vi "send and receive.vi"(6 "timeout (25000ms)":i32=25000, 8 "error in (no error)":errorcluster, 9 "data":string, 10 "command":string, 11 "daemon reference in":refnum<k5>) -> (0 "error out":errorcluster, 2 "response":string, 3 "daemon reference out":refnum<k5>)   [LabVIEW 2017]
doc: "This command is used by the API to send and receive a response from the Daemon.\n------------------------------------------\nDyLab - Network QMH Architecture 1.0.0.33\nDyson Technology Ltd Copyright (c) 2022, Dyson Technology Ltd\n____________________________________________\nDIPC 692 Daemon API 7.0.0.1\nSam Tee - Dyson Technology Ltd\nCopyright (c) 2024, Dyson Technology Ltd"
panel:
  out "Numeric":i32
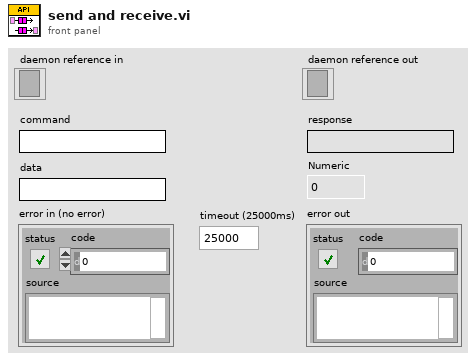
[diagram p1: front panel]
types:
  T1 = typedef "HD Config.ctl" = cluster{" PC":cluster{"PC Address":u8[], "PC Port":i32}, "FCO":cluster{"COM":refnum<visa-resource-name>, "Baudrate":u32}, "DC Power ":cluster{"COM":refnum<visa-resource-name>, "Baudrate":u32}, "PW3336":cluster{"COM":refnum<visa-resource-name>, "Baudrate":u32}, "Lefoo":cluster{"COM":refnum<visa-resource-name>, "Baudrate":u32}, "AI Model":cluster{"COM":refnum<visa-resource-name>, "Baudrate":u32}, "DIPC":cluster{"COM":refnum<visa-resource-name>}, "RFID":cluster{"IP Address":string, "Port":u16, "Retry":u16}, "Motor":cluster{"COM":refnum<visa-resource-name>, "Baudrate":u32}, "Fail_resume_mode":bool, "GRR":bool}
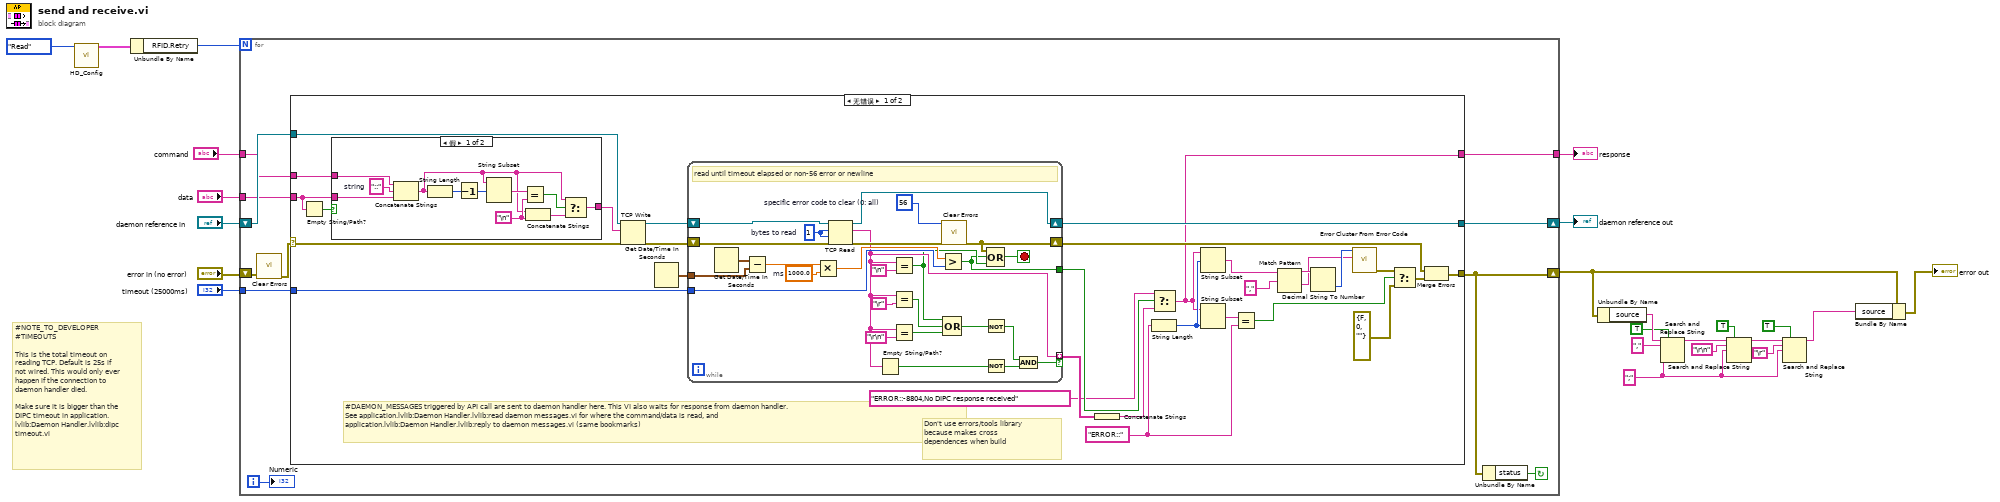
[diagram p0: block diagram]
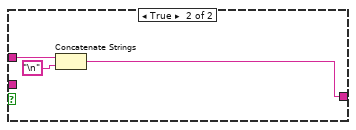
[diagram p2: hidden frame]
diagram:
  w1 = ";" ("替换字符串(\"\")")
  # "#NOTE_TO_DEVELOPER \n#TIMEOUTS\n\nThis is the total timeout on reading TCP. Default is 25s if not wired. This would only ever happen if the connection to daemon handler died.\n\nMake sure it is bigger than the DIPC timeout in application.lvlib:Daemon Handler.lvlib:dipc timeout.vi"
  n1 = call "HD_Config.vi"("Step"=enum16{"Initial", "Write", "Read"}."Read") -> ("HD Config out"=w15:T1)  [unwired: 9 in, 1 out]
  n2 = Unbundle By Name(w15) -> ("RFID.Retry"=w14:u16)
  n3 = for {
    N: w14 -> [_]
    tunnel: "data" -> [w32]
    tunnel: "timeout (25000ms)" -> [w31]
    shift-right: [w30] -> w19
    shift-left: "daemon reference in" -> [w34]
    shift-right: [w26] -> w13
    shift-left: "error in (no error)" -> [w29]
    tunnel: "command" -> [w33]
    tunnel: [w28] -> w17
    i -> [w24]
    stop <- w25 continue-if-true
    n4 = call <vilib>:"Clear Errors.vi"("error in (no error)"=w29) -> ("error out"=w27:errorcluster)  [unwired: 5 in, 1 out]
    n5 = case shown="无错误" w27 {
      selector: w27 -> [w39 w107]
      tunnel: w34 -> [w64 w106]
      tunnel: w33 -> [w61 _]
      tunnel: w32 -> [w59 _]
      tunnel: w31 -> [w56 _]
      tunnel: [w55 w106] -> w30
      tunnel: [w47 w107] -> w26
      tunnel: [w38 _] -> w28
      frame No Error {
        w50 = "ERROR::" ("t")
        # "Don't use errors/tools library\nbecause makes cross\ndependences when build"
        # "#DAEMON_MESSAGES triggered by API call are sent to daemon handler here. This VI also waits for response from daemon handler.\nSee application.lvlib:Daemon Handler.lvlib:read daemon messages.vi for where the command/data is read, and\napplication.lvlib:Daemon Handler.lvlib:reply to daemon messages.vi (same bookmarks)"
        n6 = Empty String/Path?(string/path=w59) -> (empty?=w58:bool)
        n7 = case shown="假" w58 {
          tunnel: w61 -> [w75 w78]
          tunnel: [w66 w77] -> w60
          tunnel: w59 -> [w65 _]
          frame False {
            w68 = "\n"
            w74 = "::"  # string
            n8 = Concatenate Strings(w75, w74, w65) -> (w67:string)
            n9 = String Length(string=w67) -> (length=w73:i32)
            n10 = Decrement(x=w73) -> (x-1=w72:i32)
            n11 = String Subset(string=w67, offset (0)=w72) -> (substring=w71:string)  [unwired: 1 in]
            n12 = Equal?(x=w71, y=w68) -> (x = y?=w70:bool)
            n13 = Concatenate Strings(w67, w68) -> (w69:string)
            n14 = Select(t=w67, s=w70, f=w69) -> (s? t:f=w66:string)
          }
          frame True {
            n15 = Concatenate Strings(w78, "\n") -> (w77:string)
          }
        }
        n16 = TCP Write(connection ID=w64, data in=w60, error in (no error)=w39) -> (connection ID out=w63:refnum<k5>, error out=w62:errorcluster)  [unwired: 1 in, 1 out]
        n17 = Get Date/Time In Seconds() -> (seconds since 1Jan1904=w57:timestamp)
        n18 = while {
          shift-right: [w101] -> w55
          shift-left: w63 -> [w104]
          shift-right: [w93] -> w48
          shift-left: w62 -> [w103]
          tunnel: w57 -> [w98]
          tunnel: w56 -> [w94]
          tunnel: [w84] -> w54 mode=indexing if=w81
          tunnel: [w79] -> w53
          stop <- w86 stop-if-true
          w96 = 1000.0  # ms
          w100 = 56  # specific error code to clear (0: all)
          w105 = 1  # bytes to read
          # "read until timeout elapsed or non-56 error or newline"
          n19 = Get Date/Time In Seconds() -> (seconds since 1Jan1904=w99:timestamp)
          n20 = Subtract(x=w99, y=w98) -> (x-y=w97:dbl)
          n21 = Multiply(x=w97, y=w96) -> (x*y=w95:dbl)
          n22 = TCP Read(connection ID=w104, bytes to read=w105, error in (no error)=w103, 9:w105) -> (connection ID out=w101:refnum<k5>, data out=w84:string, error out=w102:errorcluster)  [unwired: 1 in]
          n23 = Empty String/Path?(string/path=w84) -> (empty?=w83:bool)
          n24 = Equal?(x=w84, y="\n") -> (x = y?=w80:bool)
          n25 = Equal?(x=w84, y="\r") -> (x = y?=w89:bool)
          n26 = Equal?(x=w84, y="\r\n") -> (x = y?=w88:bool)
          n27 = Greater?(x=w95, y=w94) -> (0:w79:bool)
          n28 = call <vilib>:"Clear Errors.vi"("error in (no error)"=w102, "specific error code to clear (0: all)"=w100) -> ("error out"=w93:errorcluster)  [unwired: 4 in, 1 out]
          n29 = Compound Arithmetic op=OR(w80, w89, w88) -> (w87:bool)
          n30 = Not(x=w87) -> (.not. x?=w85:bool)
          n31 = Not(x=w83) -> (.not. x?=w82:bool)
          n32 = Compound Arithmetic op=OR(w93, w79, w80) -> (w86:bool)
          n33 = And(x=w85, y=w82) -> (x .and. y?=w81:bool)
        }
        n34 = Concatenate Strings(w54) -> (w52:string)
        n35 = Select(t="ERROR::-8804,No DIPC response received", s=w53, f=w52) -> (s? t:f=w38:string)
        n36 = String Length(string=w50) -> (length=w44:i32)
        n37 = String Subset(string=w38, offset (0)=w44) -> (substring=w43:string)  [unwired: 1 in]
        n38 = String Subset(string=w38, length (rest)=w44) -> (substring=w51:string)  [unwired: 1 in]
        n39 = Equal?(x=w51, y=w50) -> (x = y?=w49:bool)
        n40 = Match Pattern(string=w43, regular expression=",") -> (before substring=w41:string, after substring=w37:string)  [unwired: 1 in, 2 out]
        n41 = Decimal String To Number(string=w41) -> (number=w40:i32)  [unwired: 2 in, 1 out]
        n42 = call <vilib>:"Error Cluster From Error Code.vi"("error message (\"\")"=w37, "error code (0)"=w40) -> ("error out"=w45:errorcluster)  [unwired: 7 in]
        n43 = Select(t=w45, s=w49, f=errorcluster {"status"=FALSE, "code"=0, "source"=""} ("error constant")) -> (s? t:f=w46:errorcluster)
        n44 = Merge Errors(w48, w46) -> (w47:errorcluster)
      }
      frame Error {
      }
    }
    n45 = Unbundle By Name(w26) -> ("status"=w25:bool)
    "Numeric" <- w24
  }
  "daemon reference out" <- w19
  "response" <- w17
  n46 = Unbundle By Name(w13) -> ("source"=w11:string)
  n47 = Search and Replace String(replace all?=TRUE ("替换全部？(F)"), input string=w11, search string="," ("搜索字符串"), replace string=w1) -> (result string=w3:string)  [unwired: 4 in, 3 out]
  n48 = Search and Replace String(replace all?=TRUE ("replace all? (F)"), input string=w3, search string="\r\n", replace string=w1) -> (result string=w8:string)  [unwired: 4 in, 3 out]
  n49 = Search and Replace String(replace all?=TRUE ("replace all? (F)"), input string=w8, search string="\r", replace string=w1) -> (result string=w2:string)  [unwired: 4 in, 3 out]
  n50 = Bundle By Name(cluster=w13, "source"=w2) -> (→"error out":errorcluster)
